vi "Insert exchange into jos_modules.vi"(3 "title":string) -> ()   [LabVIEW 2010]
doc: "This example opens a connection to a database specified by the Connection string (replace the DNS name with your database) inserts a new row into the table \"myOtherTable\" (replace the SQL string with your own SQL query)."
panel:
  out "concatenated string":string
  out "error out":errorcluster
  in  "Command Text":string="INSERT INTO jos_content\n (id, title, alias, introtext, state, sectionid, mask, catid, created_by, modified, modified_by, publish_up, attribs, version, metadesc, metadata)\nVALUES ('id', 'title', 'alias', 'introtext', '1', '14', '0', '1394', '2012-12-12 12:12:12', '62', '2012-12-12 12:12:12', '62', '2012-12-12 12:12:12', 'show_title=\nlink_titles=\nshow_intro=\nshow_section=\nlink_section=\nshow_category=\nlink_category=\nshow_vote=\nshow_author=\nshow_create_date=\nshow_modify_date=\nshow_pdf_icon=\nshow_print_icon=\nshow_email_icon=\nlanguage=\nkeyref=\nreadmore=', '5', 'A book price comparison tool where 2.5% goes towards the cause! | A Student Book Project  Fundraiser', 'robots=\nauthor=');"
  in  "ConnectionString":string="DSN=stusbooks;"
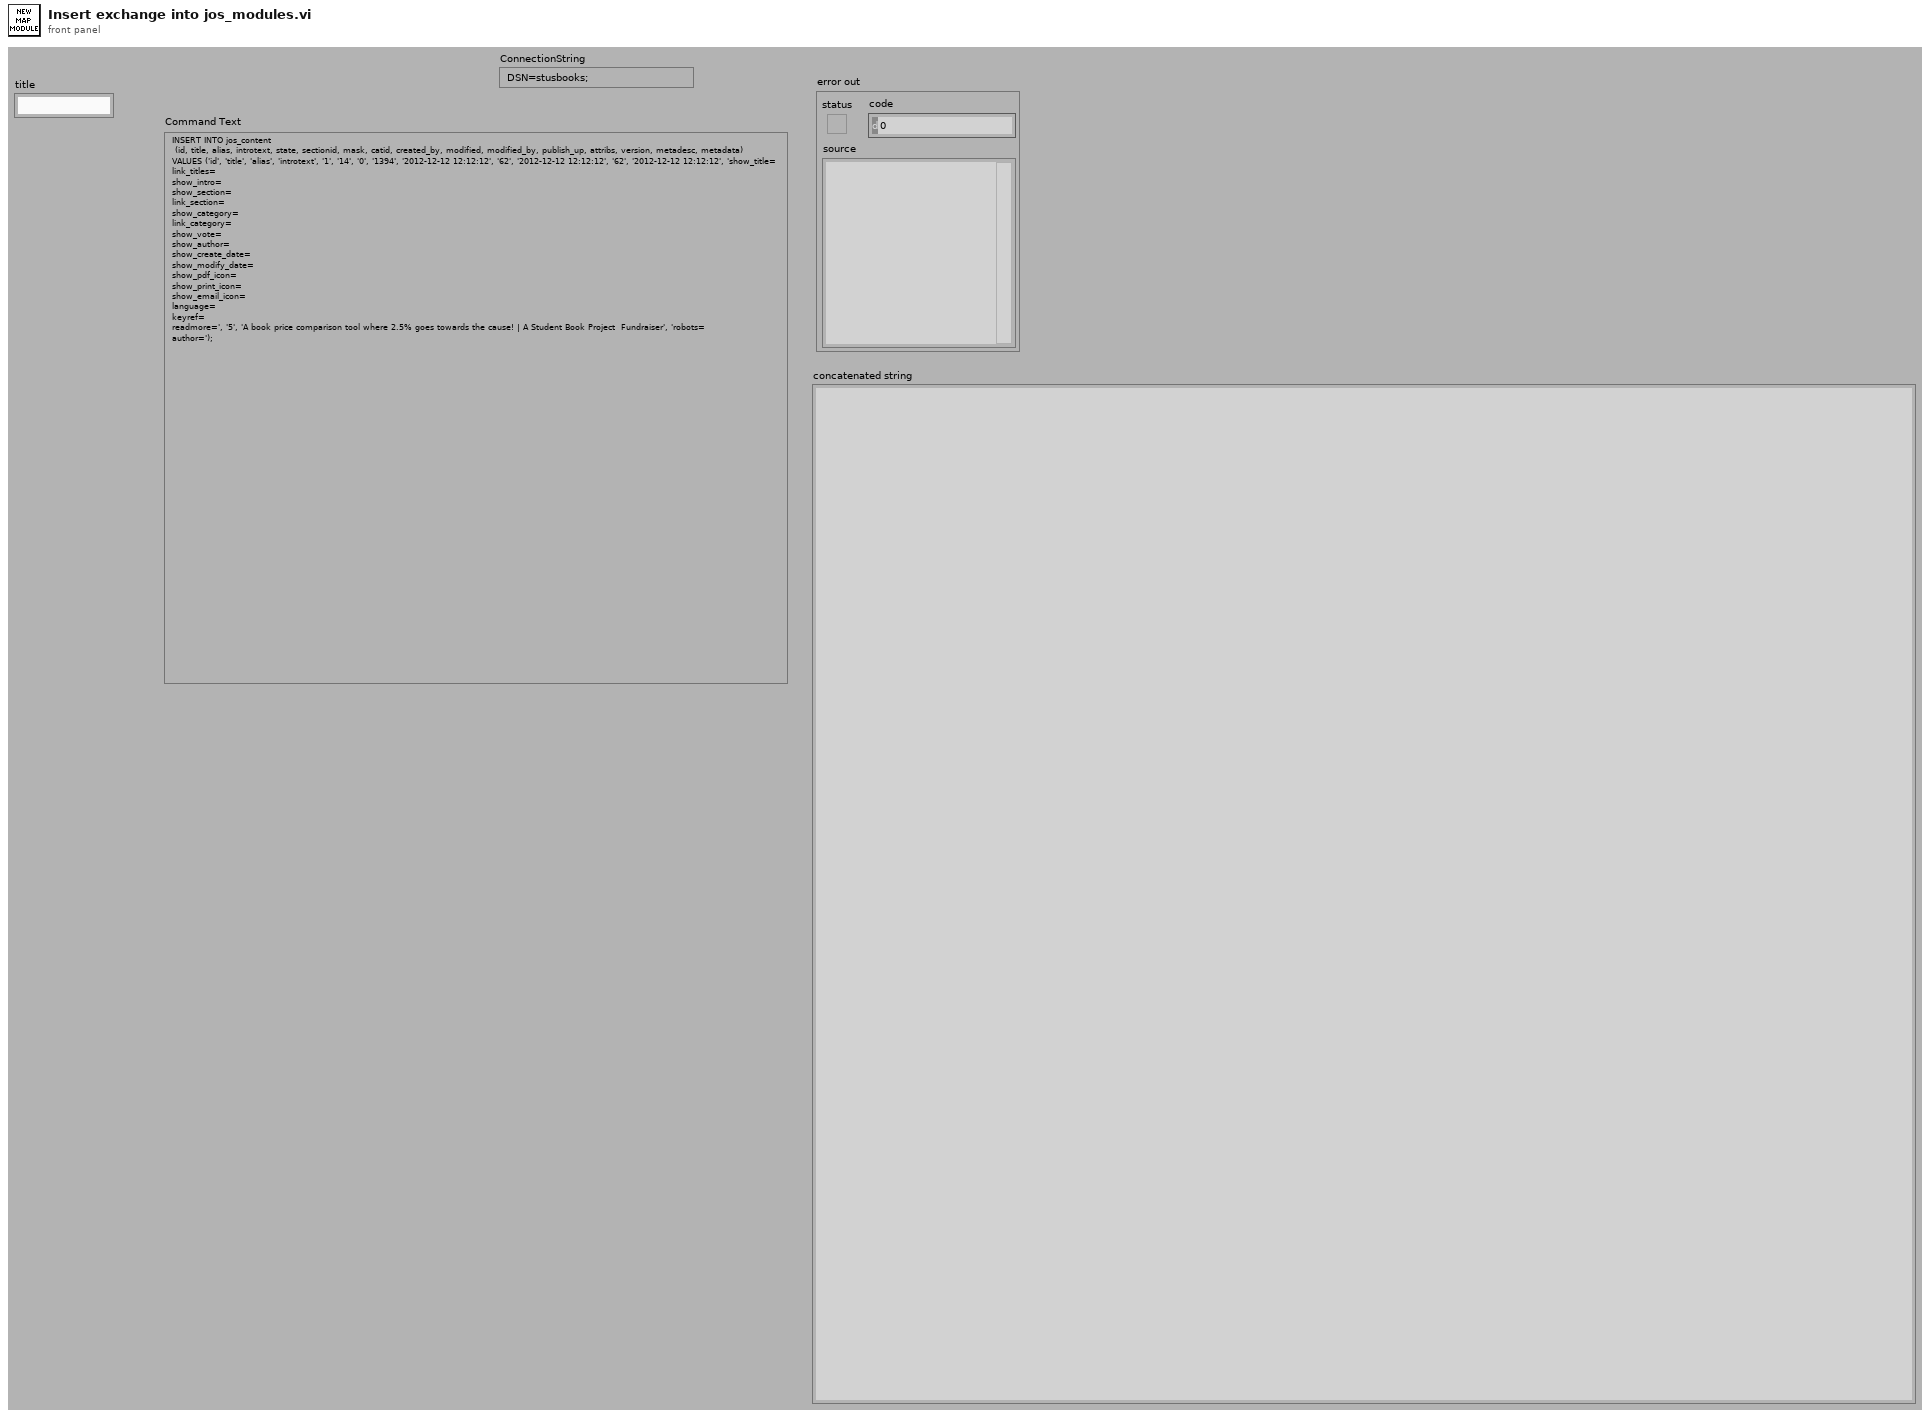
[diagram p1: front panel]
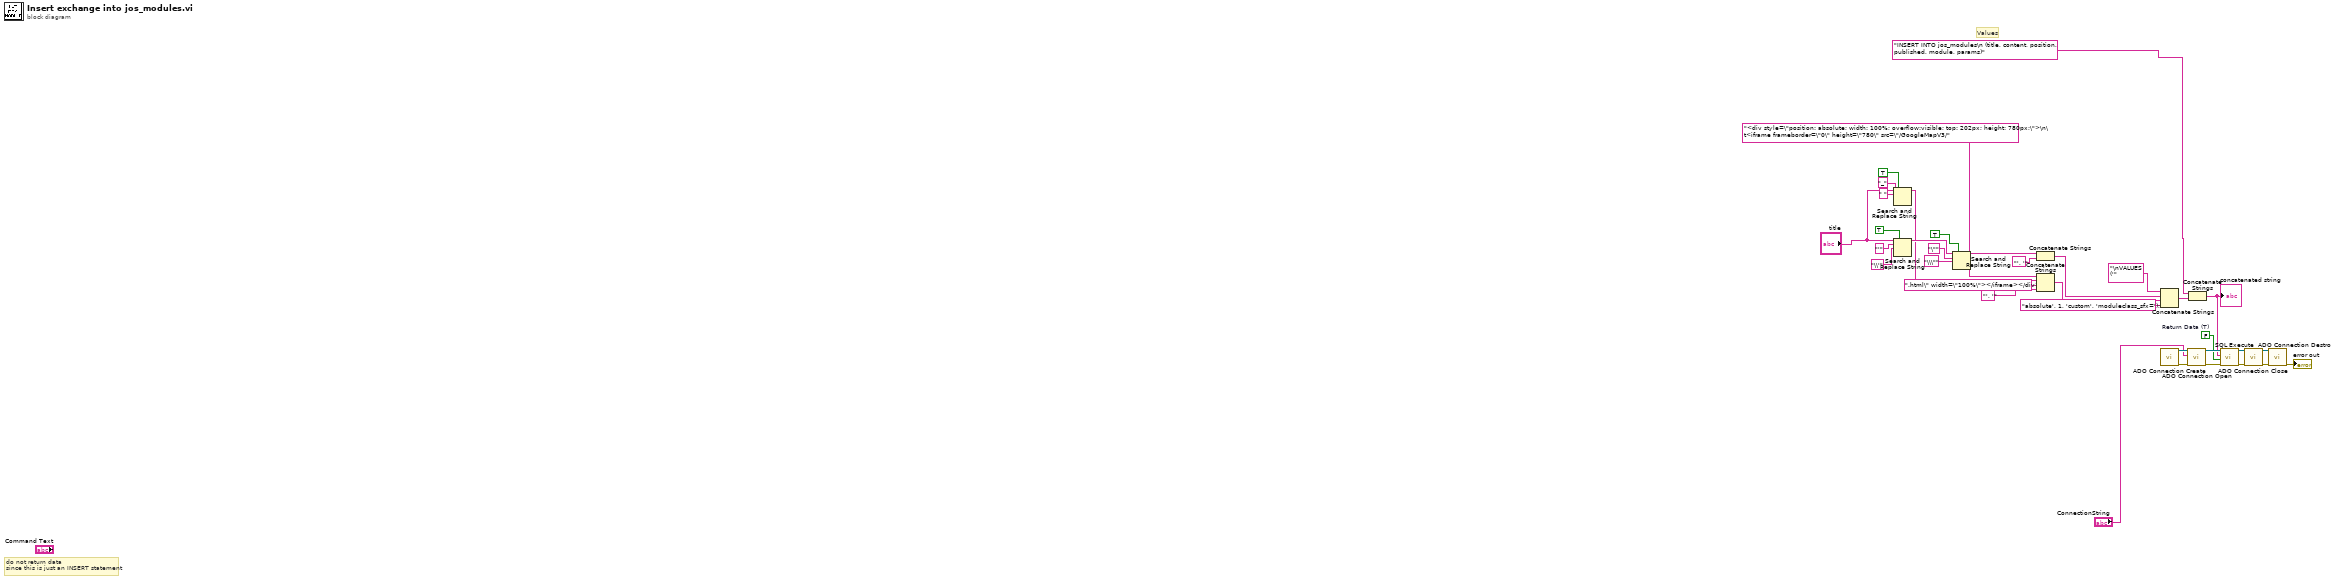
[diagram p0: block diagram]
diagram:
  w25 = FALSE  # Return Data (T)
  # "Values"
  # "do not return data\nsince this is just an INSERT statement"
  n1 = Search and Replace String(replace all?=TRUE ("replace all? (F)"), input string="title", search string=" ", replace string="_" ("replace string (\"\")")) -> (result string=w3:string)  [unwired: 4 in, 3 out]
  n2 = Search and Replace String(replace all?=TRUE ("replace all? (F)"), input string="title", search string="'", replace string="\\'" ("replace string (\"\")")) -> (result string=w19:string)  [unwired: 4 in, 3 out]
  n3 = Search and Replace String(replace all?=TRUE ("replace all? (F)"), input string=w19, search string="\"", replace string="\\\"" ("replace string (\"\")")) -> (result string=w16:string)  [unwired: 4 in, 3 out]
  n4 = Concatenate Strings(w16, "', '" ("string")) -> (w23:string)
  n5 = Concatenate Strings("<div style=\"position: absolute; width: 100%; overflow:visible; top: 202px; height: 780px;\">\n\t<iframe frameborder=\"0\" height=\"780\" src=\"/GoogleMapV3/" ("string"), w3, ".html\" width=\"100%\"></iframe></div>" ("string"), "', '" ("string")) -> (w14:string)
  n6 = Concatenate Strings("\nVALUES ('" ("string"), w23, w14, "absolute', 1, 'custom', 'moduleclass_sfx=');" ("string")) -> (w13:string)
  n7 = call "ADO Connection Create.vi"() -> ("error out"=w34:errorcluster, "ADODB._Connection Out"=w35:refnum<k7>)  [unwired: 10 in]
  n8 = call "ADO Connection Open.vi"("error in (no error)"=w34, "ConnectionString"="ConnectionString", "ADODB._Connection In"=w35) -> ("error out"=w31:errorcluster, "ADODB._Connection Out"=w32:refnum<k7>)  [unwired: 7 in]
  n9 = Concatenate Strings("INSERT INTO jos_modules\n (title, content, position, published, module, params)" ("string"), w13) -> (w12:string)
  "concatenated string" <- w12
  n10 = call "SQL Execute.vi"("error in (no error)"=w31, "Return Data (T)"=w25, "Command Text"=w12, "ADODB._Connection In"=w32) -> ("error out"=w30:errorcluster, "ADODB._Connection Out"=w29:refnum<k7>)  [unwired: 4 in, 2 out]
  n11 = call "ADO Connection Close.vi"("error in (no error)"=w30, "ADODB._Connection In"=w29) -> ("error out"=w28:errorcluster, "ADODB._Connection Out"=w27:refnum<k7>)  [unwired: 8 in]
  n12 = call "ADO Connection Destroy.vi"("error in (no error)"=w28, "ADODB._Connection In"=w27) -> ("error out"=→"error out":errorcluster)  [unwired: 9 in]
